vi "SPI Scripting.Communication FIFOs.vi"(6 "Path to SOM Engine":string="IONode\\SPIEngineSOM.vi", 7 "Path to All Nodes Resources":string="IONode\\Controls\\All Nodes Resources.ctl", 8 "error in":errorcluster, 9 "Number of SPI Devices on Bus":i32=1 min=1 step=1, 11 "Path to IO Node":path=path "D:/Documents/Projects/SPIAPI/IOEngineCode/Initialize Node Resources.vi") -> (0 "error out":errorcluster, 3 "Path to IO Node":path=path "D:/Documents/Projects/SPIAPI/IOEngineCode/Initialize Node Resources.vi")   [LabVIEW 2014, in "Initialization and IO Node Scripting.lvlib"]
uses:
  Initialization and IO Node Scripting.lvlib
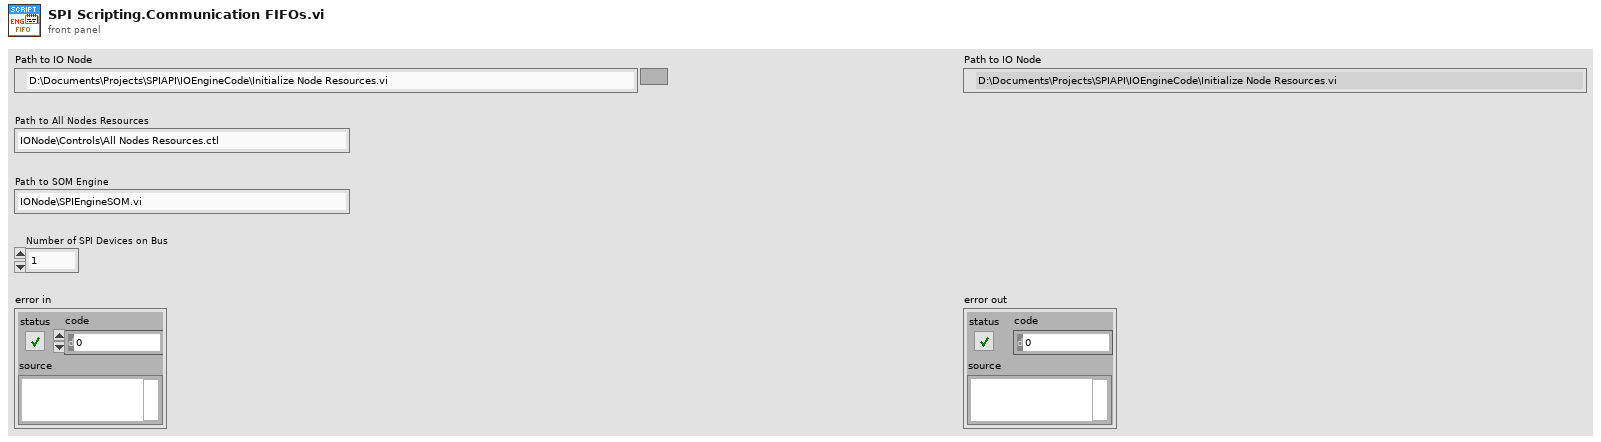
[diagram p1: front panel]
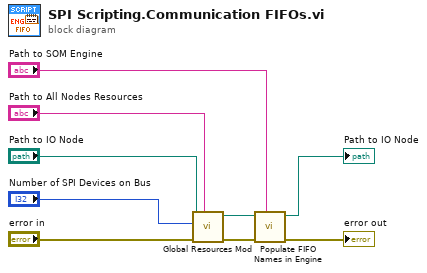
[diagram p0: block diagram]
diagram:
  n1 = call "Global Resources Mod.vi"("Path to All Nodes Resources"="Path to All Nodes Resources", "error in"="error in", "Number of SPI Devices on Bus"="Number of SPI Devices on Bus", "Path to IO Node"="Path to IO Node") -> ("error out"=w8:errorcluster, "Path to IO Node"=w9:path)  [unwired: 5 in, 1 out]
  n2 = call "Populate FIFO Names in Engine.vi"("Path to SOM Engine"="Path to SOM Engine", "error in"=w8, "Path to IO Node"=w9) -> ("error out"=→"error out":errorcluster, "Path to IO Node"=→"Path to IO Node":path)  [unwired: 7 in]
